vi "RSZVB Get Calibration Date.vi"(8 "error in (no error)":errorcluster {"code" format="%.0x"}, 10 "Channel (1)":i32=1, 11 "VISA session":refnum<visa-resource-name>) -> (0 "error out":errorcluster {"code" format="%.0x"}, 2 "Calibration Date":string, 3 "dup VISA session":refnum<visa-resource-name>)   [LabVIEW 2011]
doc: "This VI queries date and time of the channel's calibration.\n\nRemote-control command(s):\n[SENSe<Ch>:]CORRection:DATE?"
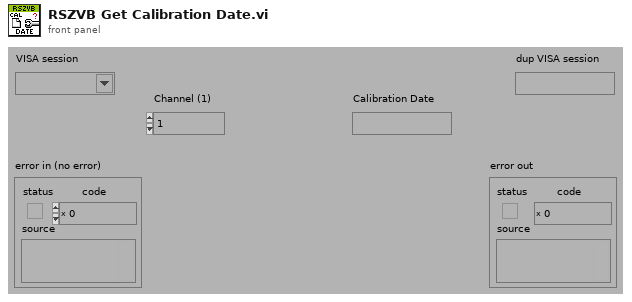
[diagram p1: front panel]
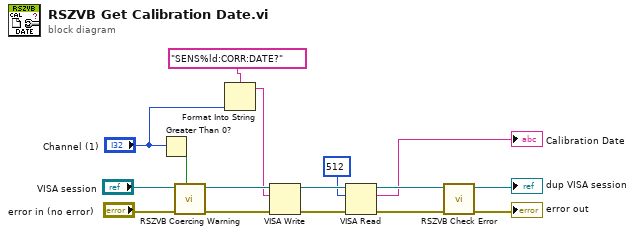
[diagram p0: block diagram]
diagram:
  n1 = Greater Than 0?(x="Channel (1)") -> (x > 0?=w4:bool)
  n2 = call "RSZVB Coercing Warning.vi"("In Range?"=w4, "error in (no error)"="error in (no error)", "VISA session"="VISA session") -> ("error out"=w15:errorcluster, "dup VISA session"=w16:refnum<visa-resource-name>)  [unwired: 7 in]
  n3 = Format Into String(format string="SENS%ld:CORR:DATE?", "Channel (1)") -> (resulting string=w1:string)  [unwired: 2 in, 1 out]
  n4 = VISA Write(VISA resource name=w16, write buffer=w1, error in (no error)=w15) -> (VISA resource name out=w14:refnum<visa-resource-name>, error out=w13:errorcluster)  [unwired: 1 out]
  n5 = VISA Read(VISA resource name=w14, byte count=u32 512 ("byte count (0)"), error in (no error)=w13) -> (VISA resource name out=w12:refnum<visa-resource-name>, read buffer=→"Calibration Date":string, error out=w11:errorcluster)  [unwired: 1 out]
  n6 = call "RSZVB Check Error.vi"("error in (no error)"=w11, "VISA session"=w12) -> ("error out"=→"error out":errorcluster, "dup VISA session"=→"dup VISA session":refnum<visa-resource-name>)  [unwired: 8 in]
